vi "PXI6514_dio.vi"() -> ()   [LabVIEW 2017]
doc: "Use this template to build a producer/consumer design pattern with events to produce queue items. Use this design pattern instead of the User Interface Event Handler pattern for user interfaces when you want to execute code asynchronously in response to an event without slowing the user interface responsiveness."
uses:
  controls/FS_PXI6514DIO.ctl
  <vilib>/DAQmx/write.llb/DAQmx Write (Digital 1D Bool 1Chan 1Samp).vi
  <vilib>/DAQmx/read.llb/DAQmx Read (Digital 1D Bool 1Chan 1Samp).vi
  <vilib>/DAQmx/write.llb/DAQmx Write (Digital Bool 1Line 1Point).vi
  <vilib>/DAQmx/create/channels.llb/DAQmx Create Channel (DO-Digital Output).vi
  <vilib>/DAQmx/miscellaneous.llb/DAQmx Fill In Error Info.vi
  <vilib>/DAQmx/create/channels.llb/DAQmx Create Channel (DI-Digital Input).vi
panel:
  out "DO_line":dbl[](array[numeric])=[0.0, 1.0, 2.0, 3.0, 4.0, 5.0, 6.0, 7.0]
  out "DI":bool[][](array[boolean])
  out "DI_line":dbl[](array[numeric])=[0.0, 1.0, 2.0, 3.0, 4.0, 5.0, 6.0, 7.0]
  in  "DO":bool[][](array[boolean])=[[FALSE, FALSE, FALSE, FALSE, FALSE, FALSE, FALSE, FALSE], [FALSE, FALSE, FALSE, FALSE, FALSE, FALSE, FALSE, FALSE], [FALSE, FALSE, FALSE, FALSE, FALSE, FALSE, FALSE, FALSE], [FALSE, FALSE, FALSE, FALSE, FALSE, FALSE, FALSE, FALSE]]
  # "PXI-651x数字状态输出/输出"
  # "Port4"
  # "Port0"
  # "Port5"
  # "Port1"
  # "Port6"
  # "Port2"
  # "Port7"
  # "Port3"
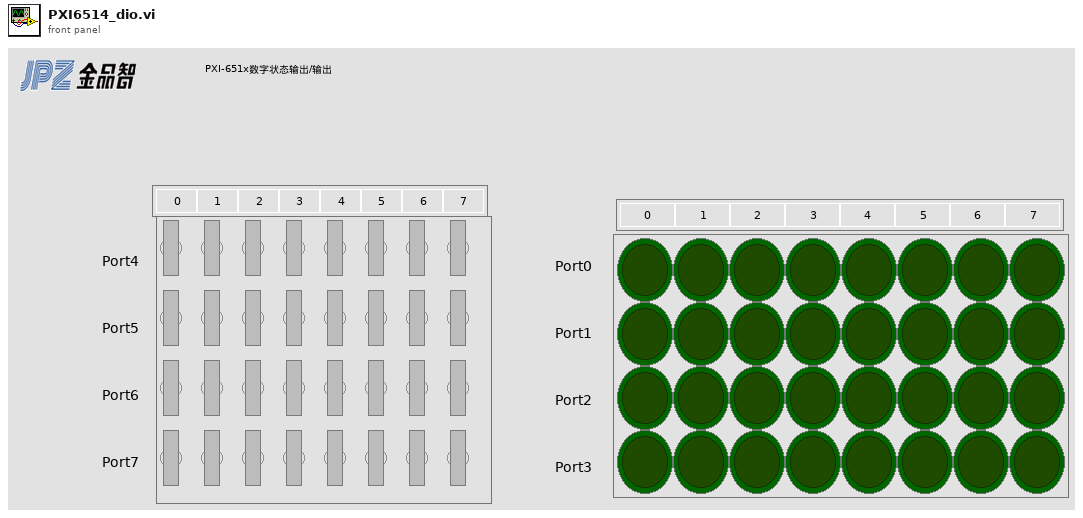
[diagram p1: front panel]
types:
  T1 = typedef "FS_PXI6514DIO.ctl" = enum16{"Initialize", "Read DI", "Write DO"}
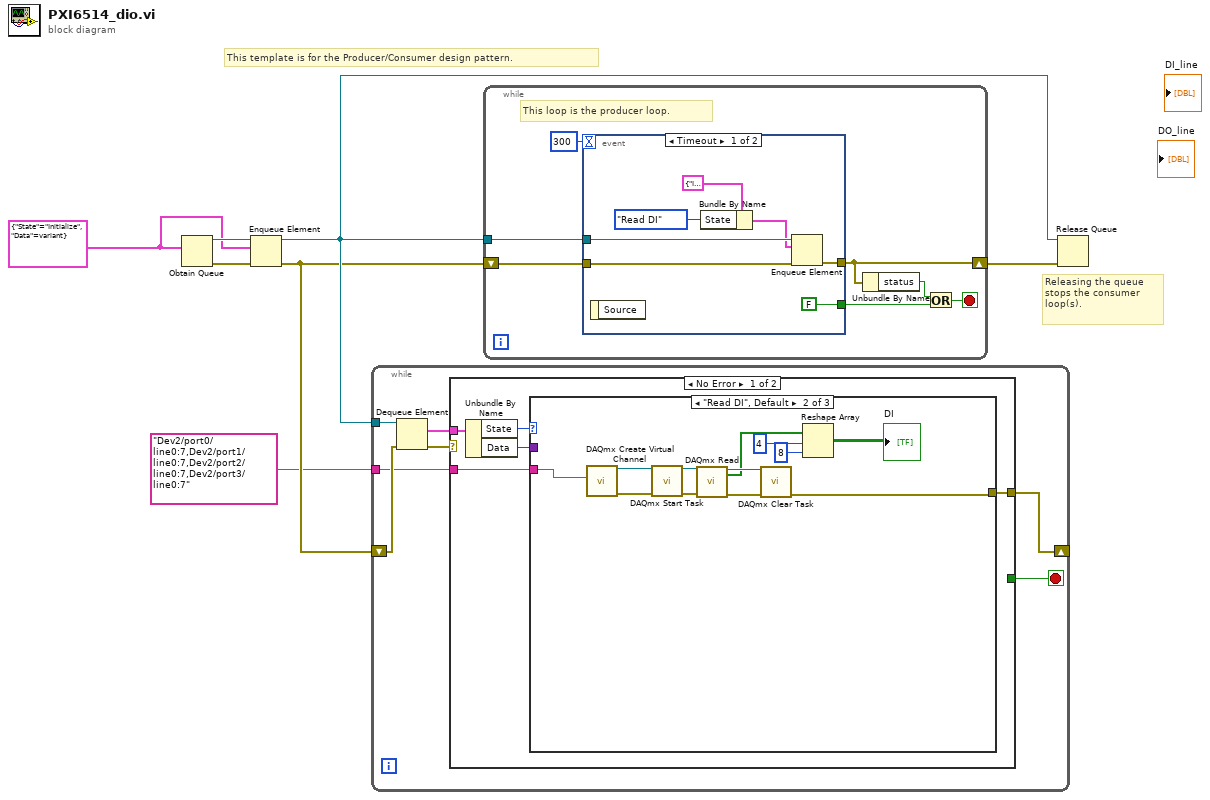
[diagram p0: block diagram]
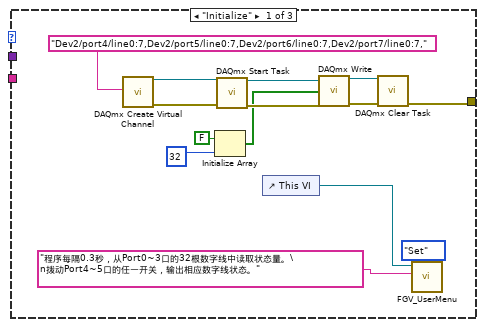
[diagram p2: hidden frame]
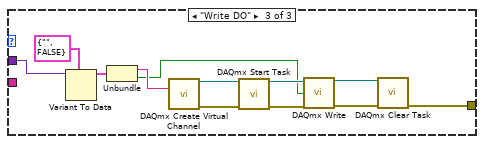
[diagram p3: hidden frame]
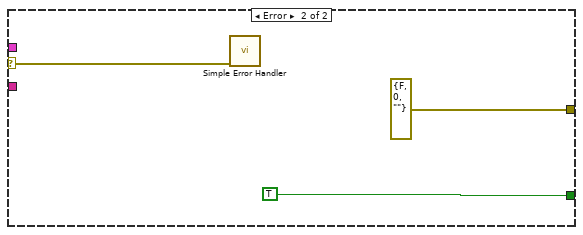
[diagram p4: hidden frame]
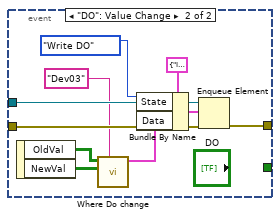
[diagram p5: hidden frame]
diagram:
  w2 = cluster{"State":T1, "Data":variant} {"State"=enum."Initialize", "Data"=variant}
  # "Releasing the queue stops the consumer loop(s)."
  # "This template is for the Producer/Consumer design pattern."
  n1 = Obtain Queue(element data type=w2) -> (queue out=w6:refnum<queue>, error out=w4:errorcluster)  [unwired: 4 in, 1 out]
  n2 = Enqueue Element(queue=w6, element=w2, error in (no error)=w4) -> (queue out=w5:refnum<queue>, error out=w3:errorcluster)  [unwired: 1 in, 1 out]
  n3 = while {
    tunnel: w5 -> [w14]
    shift-right: [w9] -> _
    shift-left: w3 -> [w10]
    tunnel: "Dev2/port0/line0:7,Dev2/port1/line0:7,Dev2/port2/line0:7,Dev2/port3/line0:7" -> [w8]
    stop <- w11 stop-if-true
    n4 = Dequeue Element(queue=w14, error in (no error)=w10) -> (element=w12:cluster{"State":T1, "Data":variant}, error out=w13:errorcluster)  [unwired: 1 in, 2 out]
    n5 = case shown="No Error" w13 {
      selector: w13 -> [_ w59]
      tunnel: w12 -> [w18 _]
      tunnel: [_ TRUE] -> w11
      tunnel: [w19 errorcluster {"status"=FALSE, "code"=0, "source"=""} ("error out")] -> w9
      tunnel: w8 -> [w15 _]
      frame No Error {
        n6 = Unbundle By Name(w18) -> ("State"=w17:T1, "Data"=w16:variant)
        n7 = case shown="\"Read DI\", Default" w17 {
          tunnel: [w33 w43 w53] -> w19
          tunnel: w16 -> [_ _ w56]
          tunnel: w15 -> [_ w38 _]
          frame "Initialize" {
            n8 = call-poly <vilib>:"DAQmx Create Virtual Channel.vi"("lines"="Dev2/port4/line0:7,Dev2/port5/line0:7,Dev2/port6/line0:7,Dev2/port7/line0:7,") -> ("task out"=w27:refnum<k21>, "error out"=w28:errorcluster)  [unwired: 13 in]
            n9 = Initialize Array(FALSE, 32) -> (w23:bool[])
            n10 = call <vilib>:"DAQmx Start Task.vi"("task/channels in"=w27, "error in"=w28) -> ("task out"=w30:refnum<k21>, "error out"=w29:errorcluster)  [unwired: 12 in]
            n11 = control-ref of="This VI"() -> (w21:refnum<vi>)
            n12 = call-poly <vilib>:"DAQmx Write.vi"("task/channels in"=w30, "data"=w23, "error in"=w29) -> ("task out"=w31:refnum<k21>, "error out"=w32:errorcluster)  [unwired: 10 in, 1 out]
            n13 = call <vilib>:"DAQmx Clear Task.vi"("task in"=w31, "error in"=w32) -> ("error out"=w33:errorcluster)  [unwired: 13 in]
            n14 = call "FGV_UserMenu.vi"("Command"=enum16{"Initialize", "Set", "Get"}."Set", "Use Info"="程序每隔0.3秒，从Port0~3口的32根数字线中读取状态量。\n拨动Port4~5口的任一开关，输出相应数字线状态。", "VI Refnum"=w21) -> ()  [unwired: 8 in, 1 out]
          }
          frame "Read DI", Default {
            n15 = call-poly <vilib>:"DAQmx Create Virtual Channel.vi"("lines"=w38) -> ("task out"=w34:refnum<k21>, "error out"=w35:errorcluster)  [unwired: 13 in]
            n16 = call <vilib>:"DAQmx Start Task.vi"("task/channels in"=w34, "error in"=w35) -> ("task out"=w37:refnum<k21>, "error out"=w36:errorcluster)  [unwired: 12 in]
            n17 = call-poly <vilib>:"DAQmx Read.vi"("task/channels in"=w37, "error in"=w36) -> ("task out"=w44:refnum<k21>, "data"=w42:bool[], "error out"=w45:errorcluster)  [unwired: 11 in]
            n18 = call <vilib>:"DAQmx Clear Task.vi"("task in"=w44, "error in"=w45) -> ("error out"=w43:errorcluster)  [unwired: 13 in]
            n19 = Reshape Array(w42, 4, 8) -> (→"DI":bool[][])
          }
          frame "Write DO" {
            n20 = Variant To Data(type=cluster{string, bool} {"", FALSE}, Variant=w56) -> (data=w54:cluster{string, bool})  [unwired: 1 in, 1 out]
            n21 = Unbundle(w54) -> (w47:string, w46:bool)
            n22 = call-poly <vilib>:"DAQmx Create Virtual Channel.vi"("lines"=w47) -> ("task out"=w49:refnum<k21>, "error out"=w48:errorcluster)  [unwired: 13 in]
            n23 = call <vilib>:"DAQmx Start Task.vi"("task/channels in"=w49, "error in"=w48) -> ("task out"=w50:refnum<k21>, "error out"=w51:errorcluster)  [unwired: 12 in]
            n24 = call-poly <vilib>:"DAQmx Write.vi"("task/channels in"=w50, "data"=w46, "error in"=w51) -> ("task out"=w52:refnum<k21>, "error out"=w57:errorcluster)  [unwired: 10 in, 1 out]
            n25 = call <vilib>:"DAQmx Clear Task.vi"("task in"=w52, "error in"=w57) -> ("error out"=w53:errorcluster)  [unwired: 13 in]
          }
        }
      }
      frame Error {
        n26 = call <vilib>:"Simple Error Handler.vi"("error in (no error)"=w59) -> ()  [unwired: 4 in, 5 out]
      }
    }
  }
  n27 = while {
    shift-right: [w63] -> w7
    shift-left: w3 -> [w66]
    tunnel: w5 -> [w67]
    stop <- w64 stop-if-true
    # "This loop is the producer loop."
    n28 = event shown="[0] Timeout" {
      selector: _ -> [_ _]
      dyn-events: _ -> [_ _]
      timeout: 300 -> [_ _]
      tunnel: w67 -> [w74 w82]
      tunnel: w66 -> [w73 w84]
      tunnel: [w72 w83] -> w63
      tunnel: [FALSE _] -> w65
      event Timeout {
        n29 = event-data() -> ()  [unwired: 1 in, 1 out]
        n30 = Bundle By Name(cluster=cluster{"State":T1, "Data":variant} {"State"=enum."Initialize", "Data"=variant}, "State"=FS_PXI6514DIO."Read DI" ("element")) -> (w68:cluster{"State":T1, "Data":variant})
        n31 = Enqueue Element(queue=w74, element=w68, error in (no error)=w73) -> (error out=w72:errorcluster)  [unwired: 1 in, 2 out]
      }
      event "DO": Value Change {
        n32 = event-data() -> ("OldVal"=w80:bool[][], "NewVal"=w81:bool[][])  [unwired: 1 in]
        n33 = call "Where Do change.vi"("Device Name"="Dev03", "New Value"=w81, "Old Value"=w80) -> ("Out_prar"=w76:cluster{"Channel":string, "New_V":bool})  [unwired: 8 in]
        n34 = Bundle By Name(cluster=cluster{"State":T1, "Data":variant} {"State"=enum."Initialize", "Data"=variant}, "State"=FS_PXI6514DIO."Write DO", "Data"=w76) -> (w77:cluster{"State":T1, "Data":variant})
        n35 = Enqueue Element(queue=w82, element=w77, error in (no error)=w84) -> (error out=w83:errorcluster)  [unwired: 1 in, 2 out]
      }
    }
    n36 = Unbundle By Name(w63) -> ("status"=w62:bool)
    n37 = Or(x=w62, y=w65) -> (x .or. y?=w64:bool)
  }
  n38 = Release Queue(queue=w5, error in (no error)=w7) -> ()  [unwired: 1 in, 3 out]
